vi "Battery_Charger_green_batteries.vi"() -> ()   [LabVIEW 2015]
uses:
  Battery_Charger_variables.vi
  <vilib>/Utility/NIReport.llb/NI_report.lvclass
  <instrlib>/Agilent N6700 Series/Agilent N6700 Series.lvlib
  <vilib>/addons/_office/NI_ReportGenerationToolkit.lvlib
panel:
  in  "Negative Voltage Limit (0.0 volts)":dbl format="%^.3e"
  in  "Positive Voltage Limit  (5.0 V)":dbl=5.0 format="%^.3e"
  in  "Channel Name (1)":string="4"
  in  "VISA resource name":refnum<visa-resource-name>="USB0::0x0957::0x0F07::MY53002228::INSTR"
  out "Charged":bool
  in  "Stop":bool
  out "Voltage Graph":dbl[](graph)
  out "Voltage Measurement":dbl format="%^.3e"
  out "Current Measurement":dbl format="%^.3e"
  out "Count":i32
  out "Current Graph":dbl[](graph)
  in  "report file path":path=path "C:/Users/Tulio/Documents/LabView Projects/Battery_Charger_Green_Batteries/Battery_Charger.xlsx"
  in  "Start":bool
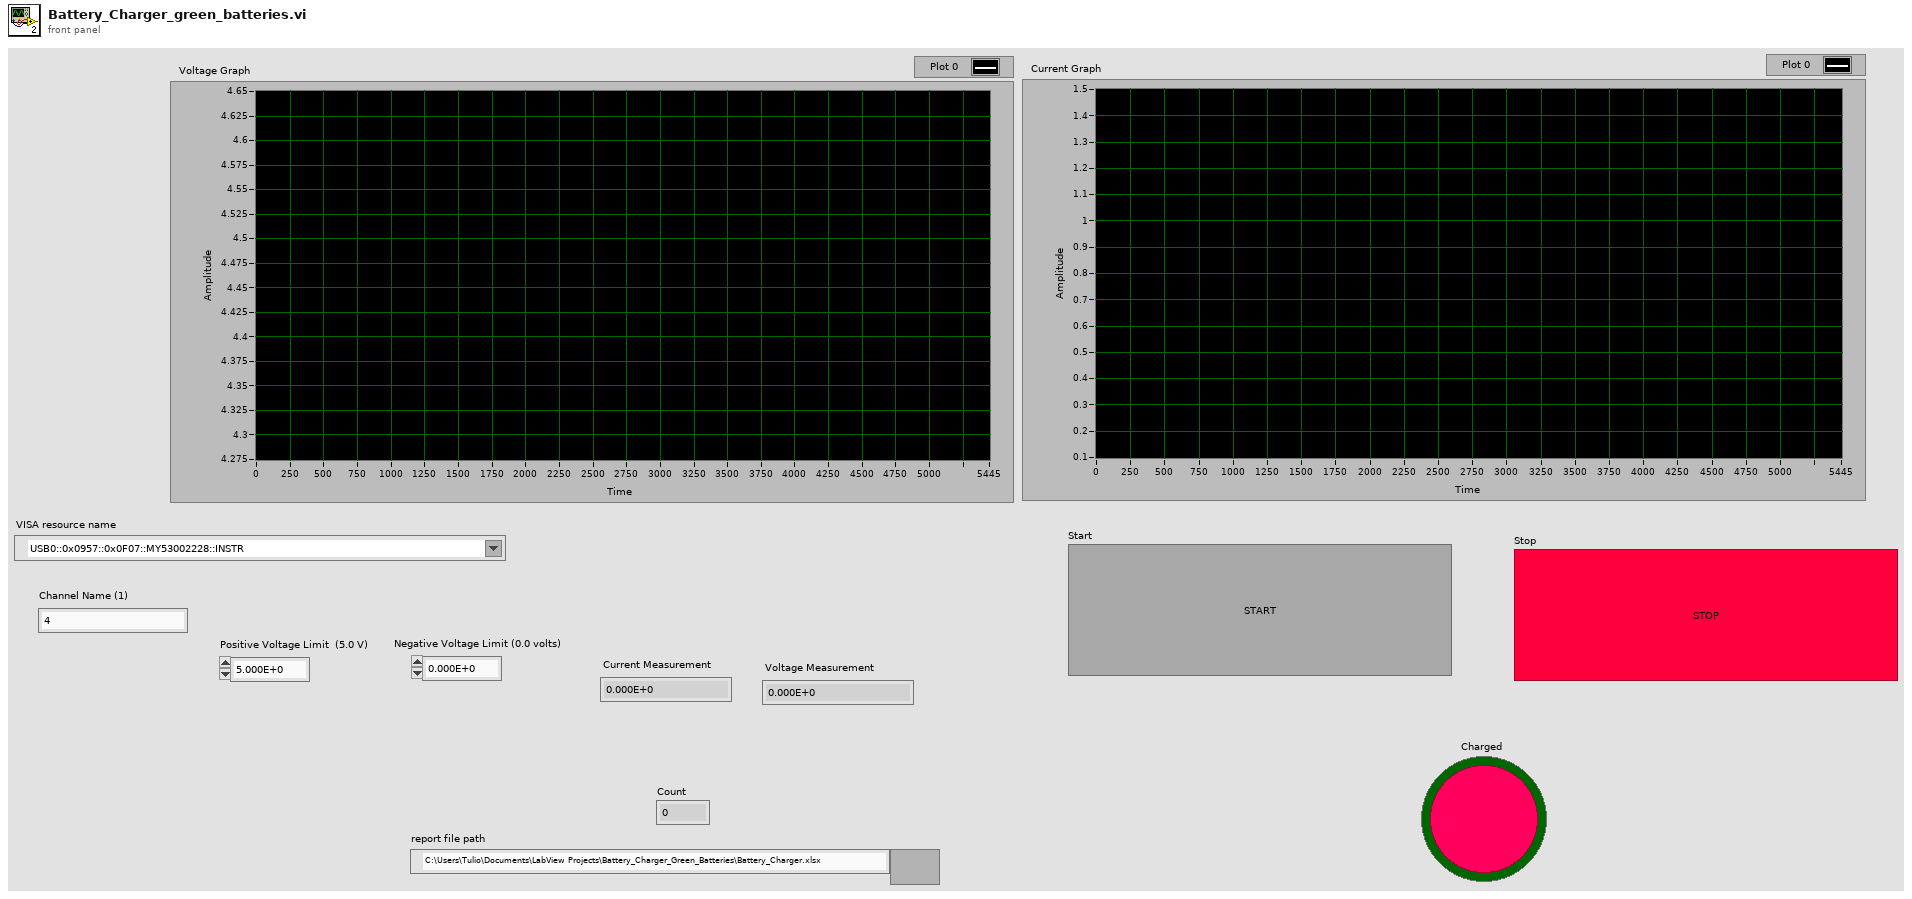
[diagram p1: front panel]
types:
  T1 = enum16{"Standard Report", "HTML", "Word", "Excel"}
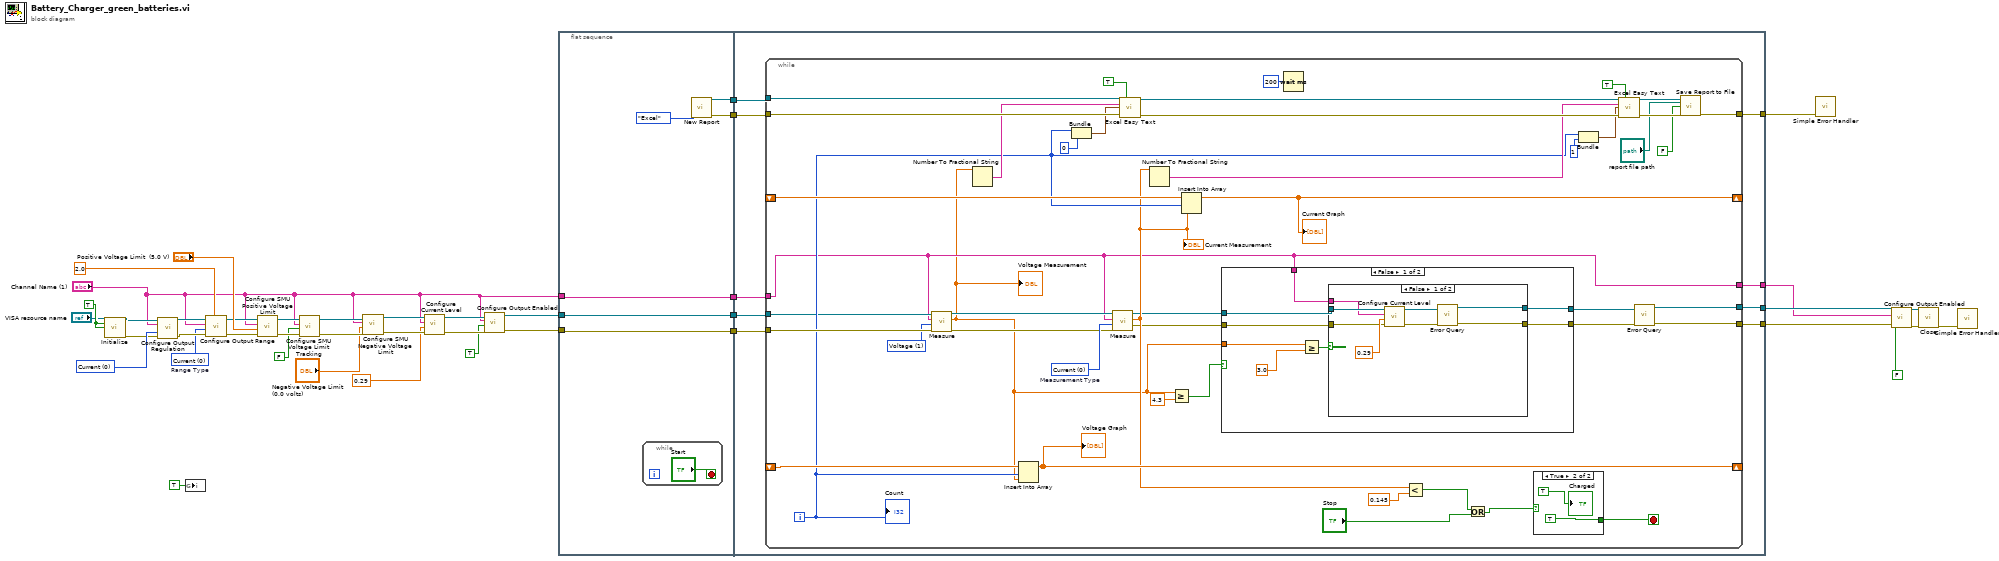
[diagram p0: block diagram]
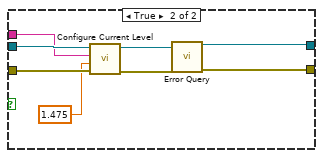
[diagram p2: hidden frame]
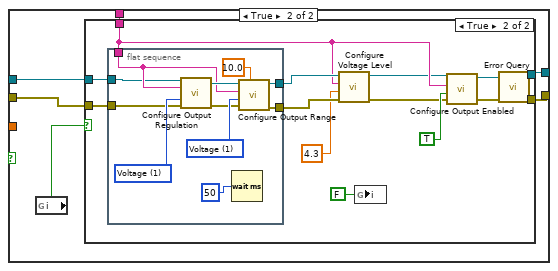
[diagram p3: hidden frame]
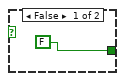
[diagram p5: hidden frame]
diagram:
  w25 = 0 items=["Voltage"=1, "Current"=0] ("Priority (1: Voltage)")
  w28 = TRUE ("Reset? (T: Yes)")
  w27 = 0 items=["Voltage"=1, "Current"=0]  # Range Type
  n1 = call <instrlib>:"Initialize.vi"("VISA resource name"="VISA resource name", "ID Query? (T: Yes)"=w28, "Reset? (T: Yes)"=w28) -> ("VISA resource name out"=w17:refnum<visa-resource-name>, "error out"=w16:errorcluster)  [unwired: 11 in]
  n2 = call <instrlib>:"Configure Output Regulation.vi"("VISA resource name"=w17, "Channel Name (1)"="Channel Name (1)", "Output Regulation Priority (1: Voltage)"=w25, "error in (no error)"=w16) -> ("VISA resource name out"=w29:refnum<visa-resource-name>, "error out"=w30:errorcluster)  [unwired: 10 in]
  n3 = global write "Battery_Charger_variables.vi" "i"(TRUE ("i")) -> ()
  n4 = call <instrlib>:"Configure Output Range.vi"("Range (0.0)"=2.0, "error in (no error)"=w30, "Range Type (1: Voltage)"=w27, "Channel Name (1)"="Channel Name (1)", "VISA resource name"=w29) -> ("error out"=w32:errorcluster, "VISA resource name out"=w31:refnum<visa-resource-name>)  [unwired: 5 in]
  n5 = call <instrlib>:"Configure SMU Positive Voltage Limit.vi"("error in (no error)"=w32, "Positive Voltage Limit (0.0 volts)"="Positive Voltage Limit  (5.0 V)", "Channel Name (1)"="Channel Name (1)", "VISA resource name"=w31) -> ("error out"=w34:errorcluster, "VISA resource name out"=w33:refnum<visa-resource-name>)  [unwired: 6 in]
  n6 = call <instrlib>:"Configure SMU Voltage Limit Tracking.vi"("error in (no error)"=w34, "Enable Voltage Limit Tracking (False)"=FALSE, "Channel Name (1)"="Channel Name (1)", "VISA resource name"=w33) -> ("error out"=w21:errorcluster, "VISA resource name out"=w22:refnum<visa-resource-name>)  [unwired: 6 in]
  n7 = call <instrlib>:"Configure SMU Negative Voltage Limit.vi"("error in (no error)"=w21, "Negative Voltage Limit (0.0 volts)"="Negative Voltage Limit (0.0 volts)", "Channel Name (1)"="Channel Name (1)", "VISA resource name"=w22) -> ("error out"=w18:errorcluster, "VISA resource name out"=w19:refnum<visa-resource-name>)  [unwired: 6 in]
  n8 = call <instrlib>:"Configure Current Level.vi"("error in (no error)"=w18, "Level  (0.0 A)"=0.29, "Channel Name (1)"="Channel Name (1)", "VISA resource name"=w19) -> ("error out"=w37:errorcluster, "VISA resource name out"=w38:refnum<visa-resource-name>)  [unwired: 6 in]
  n9 = call <instrlib>:"Configure Output Enabled.vi"("error in (no error)"=w37, "Enable Output (False)"=TRUE, "Channel Name (1)"="Channel Name (1)", "VISA resource name"=w38) -> ("error out"=w12:errorcluster, "VISA resource name out"=w13:refnum<visa-resource-name>)  [unwired: 6 in]
  n10 = flat-sequence {
    tunnel: [w42] -> w41
    tunnel: [w46] -> w40
    tunnel: [w45] -> w39
    tunnel: w13 -> [w44]
    tunnel: w12 -> [w43]
    tunnel: [w44] -> w11
    tunnel: [w43] -> w10
    tunnel: "Channel Name (1)" -> [w42]
    tunnel: w41 -> [w57]
    tunnel: w40 -> [w54]
    tunnel: w39 -> [w53]
    tunnel: w11 -> [w56]
    tunnel: w10 -> [w55]
    tunnel: [w52] -> w4
    tunnel: [w51] -> w3
    tunnel: [w50] -> w2
    tunnel: [w49] -> w1
    frame #0 {
      n11 = while {
        stop <- "Start" stop-if-true
      }
      n12 = call <vilib>:"New Report.vi"("report type"=T1."Excel") -> ("report out"=w46:refnum<class "NI_report.lvclass">, "error out"=w45:errorcluster)  [unwired: 13 in]
    }
    frame #1 {
      n13 = while {
        tunnel: w57 -> [w59]
        tunnel: w56 -> [w69]
        tunnel: w55 -> [w78]
        tunnel: [w87] -> w52
        tunnel: [w88] -> w51
        tunnel: [w59] -> w50
        tunnel: w54 -> [w100]
        tunnel: w53 -> [w99]
        tunnel: [w84] -> w49
        shift-right: [w90] -> _
        shift-left: _ -> [w89]
        shift-right: [w73] -> _
        shift-left: _ -> [w75]
        i -> [w74]
        stop <- w101 stop-if-true
        w77 = 1 items=["Current", "Voltage", "Power"] ("Measurement Type (1: Voltage)")
        w102 = 0 items=["Voltage"=1, "Current"=0]  # Measurement Type
        n14 = call <instrlib>:"Measure.vi"("error in (no error)"=w78, "Measurement Type (1: Voltage)"=w77, "Channel Name (1)"=w59, "VISA resource name"=w69) -> ("error out"=w80:errorcluster, "Measurement"=w58:dbl, "VISA resource name out"=w79:refnum<visa-resource-name>)  [unwired: 5 in]
        "Voltage Measurement" <- w58
        n15 = Number To Fractional String(number=w58) -> (F-format string=w76:string)  [unwired: 3 in]
        n16 = Insert Into Array(array=w75, index=w74, new element=w58) -> (w73:dbl[])
        "Voltage Graph" <- w73
        n17 = Bundle(w74, "offset (0)"=0) -> (w98:cluster{i32, "offset (0)":i32})  [unwired: 1 in]
        n18 = call <instrlib>:"Measure.vi"("error in (no error)"=w80, "Measurement Type (1: Voltage)"=w102, "Channel Name (1)"=w59, "VISA resource name"=w79) -> ("error out"=w62:errorcluster, "Measurement"=w67:dbl, "VISA resource name out"=w63:refnum<visa-resource-name>)  [unwired: 5 in]
        "Current Measurement" <- w67
        n19 = call <vilib>:"Excel Easy Text.vi"("report in"=w100, "border? (F)"=TRUE, "text"=w76, "start (-1, -1)"=w98, "error in (no error)"=w99) -> ("report out"=w95:refnum<class "NI_report.lvclass">, "error out"=w96:errorcluster)  [unwired: 6 in, 3 out]
        n20 = Number To Fractional String(number=w67) -> (F-format string=w92:string)  [unwired: 3 in]
        n21 = Greater Or Equal?(x=w58, y=4.3) -> (x >= y?=w65:bool)
        n22 = Insert Into Array(array=w89, index=w74, new element=w67) -> (w90:dbl[])
        "Current Graph" <- w90
        n23 = case shown="False" w65 {
          tunnel: w63 -> [w107 w129]
          tunnel: w62 -> [w106 w128]
          tunnel: w59 -> [w105 w130]
          tunnel: [w104 w131] -> w61
          tunnel: [w103 w132] -> w60
          tunnel: w58 -> [w109 _]
          frame False {
            n24 = Greater Or Equal?(x=w109, y=3.0) -> (x >= y?=w110:bool)
            n25 = case shown="False" w110 {
              tunnel: w107 -> [w114 w126]
              tunnel: w106 -> [w115 w125]
              tunnel: w105 -> [w113 w124]
              tunnel: [w112 w121] -> w104
              tunnel: [w111 w120] -> w103
              frame False {
                n26 = call <instrlib>:"Configure Current Level.vi"("error in (no error)"=w115, "Level  (0.0 A)"=0.29, "Channel Name (1)"=w113, "VISA resource name"=w114) -> ("error out"=w117:errorcluster, "VISA resource name out"=w118:refnum<visa-resource-name>)  [unwired: 6 in]
                n27 = call <instrlib>:"Error Query.vi"("VISA resource name"=w118, "error in (no error)"=w117) -> ("VISA resource name out"=w112:refnum<visa-resource-name>, "error out"=w111:errorcluster)  [unwired: 10 in, 2 out]
              }
              frame True {
                n28 = call <instrlib>:"Configure Current Level.vi"("error in (no error)"=w125, "Level  (0.0 A)"=1.475, "Channel Name (1)"=w124, "VISA resource name"=w126) -> ("error out"=w122:errorcluster, "VISA resource name out"=w123:refnum<visa-resource-name>)  [unwired: 6 in]
                n29 = call <instrlib>:"Error Query.vi"("VISA resource name"=w123, "error in (no error)"=w122) -> ("VISA resource name out"=w121:refnum<visa-resource-name>, "error out"=w120:errorcluster)  [unwired: 10 in, 2 out]
              }
            }
          }
          frame True {
            n30 = global read "Battery_Charger_variables.vi" "i"() -> (w127:bool)
            n31 = case shown="True" w127 {
              tunnel: [w133 w146] -> w132
              tunnel: [w134 w145] -> w131
              tunnel: w130 -> [_ w140]
              tunnel: w129 -> [w134 w137]
              tunnel: w128 -> [w133 w136]
              frame False {
              }
              frame True {
                n32 = flat-sequence {
                  tunnel: w140 -> [w156]
                  tunnel: [w155] -> w142
                  tunnel: [w154] -> w143
                  tunnel: w137 -> [w152]
                  tunnel: w136 -> [w151]
                  frame #0 {
                    w157 = 1 items=["Voltage"=1, "Current"=0] ("Range Type (1: Voltage)")
                    w158 = 1 items=["Voltage"=1, "Current"=0] ("Output Regulation Priority (1: Voltage)")
                    n33 = call <instrlib>:"Configure Output Regulation.vi"("VISA resource name"=w152, "Channel Name (1)"=w156, "Output Regulation Priority (1: Voltage)"=w158, "error in (no error)"=w151) -> ("VISA resource name out"=w159:refnum<visa-resource-name>, "error out"=w150:errorcluster)  [unwired: 10 in]
                    n34 = Wait (ms)(milliseconds to wait=u32 50) -> ()  [unwired: 1 out]
                    n35 = call <instrlib>:"Configure Output Range.vi"("Range (0.0)"=10.0, "error in (no error)"=w150, "Range Type (1: Voltage)"=w157, "Channel Name (1)"=w156, "VISA resource name"=w159) -> ("error out"=w154:errorcluster, "VISA resource name out"=w155:refnum<visa-resource-name>)  [unwired: 5 in]
                  }
                }
                n36 = call <instrlib>:"Configure Voltage Level.vi"("error in (no error)"=w143, "Level  (0.0 volts)"=4.3, "Channel Name (1)"=w140, "VISA resource name"=w142) -> ("error out"=w138:errorcluster, "VISA resource name out"=w139:refnum<visa-resource-name>)  [unwired: 6 in]
                n37 = global write "Battery_Charger_variables.vi" "i"(FALSE ("i")) -> ()
                n38 = call <instrlib>:"Configure Output Enabled.vi"("error in (no error)"=w138, "Enable Output (False)"=TRUE, "Channel Name (1)"=w140, "VISA resource name"=w139) -> ("error out"=w147:errorcluster, "VISA resource name out"=w148:refnum<visa-resource-name>)  [unwired: 6 in]
                n39 = call <instrlib>:"Error Query.vi"("VISA resource name"=w148, "error in (no error)"=w147) -> ("VISA resource name out"=w145:refnum<visa-resource-name>, "error out"=w146:errorcluster)  [unwired: 10 in, 2 out]
              }
            }
          }
        }
        n40 = Wait (ms)(milliseconds to wait=u32 200) -> ()  [unwired: 1 out]
        n41 = Less?(x=w67, y=0.145) -> (x < y?=w68:bool)
        n42 = Or(x=w68, y="Stop") -> (x .or. y?=w71:bool)
        n43 = case shown="True" w71 {
          tunnel: [FALSE TRUE ("stop")] -> w101
          frame False {
          }
          frame True {
            "Charged" <- TRUE
          }
        }
        n44 = Bundle(w74, "offset (0)"=1) -> (w93:cluster{i32, "offset (0)":i32})  [unwired: 1 in]
        n45 = call <vilib>:"Excel Easy Text.vi"("report in"=w95, "border? (F)"=TRUE, "text"=w92, "start (-1, -1)"=w93, "error in (no error)"=w96) -> ("report out"=w86:refnum<class "NI_report.lvclass">, "error out"=w85:errorcluster)  [unwired: 6 in, 3 out]
        n46 = call <instrlib>:"Error Query.vi"("VISA resource name"=w61, "error in (no error)"=w60) -> ("VISA resource name out"=w88:refnum<visa-resource-name>, "error out"=w87:errorcluster)  [unwired: 10 in, 2 out]
        n47 = call-dynamic "Save Report to File.vi"("report in"=w86, "report file path"="report file path", "prompt to replace? (F)"=FALSE, "error in (no error)"=w85) -> ("error out"=w84:errorcluster)  [unwired: 10 in, 1 out]
        "Count" <- w74
      }
    }
  }
  n48 = call <vilib>:"Simple Error Handler.vi"("error in (no error)"=w1) -> ()  [unwired: 1 in, 8 out]
  n49 = call <instrlib>:"Configure Output Enabled.vi"("error in (no error)"=w4, "Enable Output (False)"=FALSE, "Channel Name (1)"=w2, "VISA resource name"=w3) -> ("error out"=w6:errorcluster, "VISA resource name out"=w7:refnum<visa-resource-name>)  [unwired: 6 in]
  n50 = call <instrlib>:"Close.vi"("VISA resource name"=w7, "error in (no error)"=w6) -> ("error out"=w8:errorcluster)  [unwired: 13 in]
  n51 = call <vilib>:"Simple Error Handler.vi"("error in (no error)"=w8) -> ()  [unwired: 4 in, 5 out]
